vi "Control_Panel_Execute.vi"() -> ()   [LabVIEW 2019]
uses:
  Globals/Control_Panel_Globals.vi
  <vilib>/Rock Robotics/WPI/ThirdParty/REV Robotics/SPARK MAX/Typedef/Spark MAX Control Type.ctl
panel:
  in  "Positional Throttle":dbl
  in  "Color Input From Our Sensor":enum16{"Yellow", "Red", "Green", "Blue"}(ring)
  in  "time_to_run":u32
  in  "Rotational Throttle":dbl
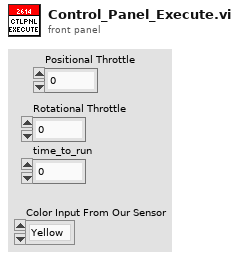
[diagram p1: front panel]
types:
  T1 = typedef "WPI_MotorControlDeviceRef.ctl" = cluster{"DeviceStatus":errorcluster, "Type":T2, "PWM":cluster{"PWM Channel":T3, "DeadBand":T4}, "CAN":cluster{"Device Number":u8, "SetOutput VI Ref":variant, "GetOutput VI Ref":variant, "Enable VI Ref":variant, "Disable VI Ref":variant, "Data":variant}, "Invert":bool, "DIO PWM":cluster{"PWM \"Enable\" Channel":T3, "DIOChannel":T5, "PWM Rate":dbl}}
  T2 = typedef "WPI_MotorControlType.ctl" = enum16{"PWM", "CAN", "DIO PWM"}
  T3 = typedef "FPGA_DIOPWMChannel.ctl" = enum8{"PWM 0", "PWM 1", "PWM 2", "PWM 3", "PWM 4", "PWM 5", "PWM 6", "PWM 7", "PWM 8", "PWM 9", "PWM MXP 0", "PWM MXP 1", "PWM MXP 2", "PWM MXP 3", "PWM MXP 4", "PWM MXP 5", "PWM MXP 6", "PWM MXP 7", "PWM MXP 8", "PWM MXP 9", "Invalid"}
  T4 = typedef "WPI_PWMDeadband.ctl" = cluster{"Name":string, "maxPositivePwm":i32, "minPositivePwm":i32, "centerPwm":i32, "maxNegativePwm":i32, "minNegativePwm":i32, "angularRange":u16}
  T5 = typedef "FPGA_DIOChannel.ctl" = enum8{"DIO 0", "DIO 1", "DIO 2", "DIO 3", "DIO 4", "DIO 5", "DIO 6", "DIO 7", "DIO 8", "DIO 9", "DIO MXP 0", "DIO MXP 1", "DIO MXP 2", "DIO MXP 3", "DIO MXP 4", "DIO MXP 5", "DIO MXP 6", "DIO MXP 7", "DIO MXP 8", "DIO MXP 9", "DIO MXP 10", "DIO MXP 11", "DIO MXP 12", "DIO MXP 13", "DIO MXP 14", "DIO MXP 15", "SPI Port CS1", "SPI Port CS2", "SPI Port CS3", "SPI Port MISO", "SPI Port MOSI", "Invalid"}
  T6 = typedef "Spark MAX Control Type.ctl" = enum16{"Percent VBus", "Voltage", "Velocity", "Position", "Smart Motion", "Current", "Smart Velocity"}
  T7 = typedef "Control_Panel_Cluster.ctl" = cluster{"Control_State":T8, "Start_Movement":bool, "Abort":bool, "Rotation_Control?":bool, "Positional_Control? ":bool, "Throttle":dbl}
  T8 = typedef "Control_Panel_States.ctl" = enum16{"No-Op", "Rotational_Control", "Positional_Control", "Manual_Control"}
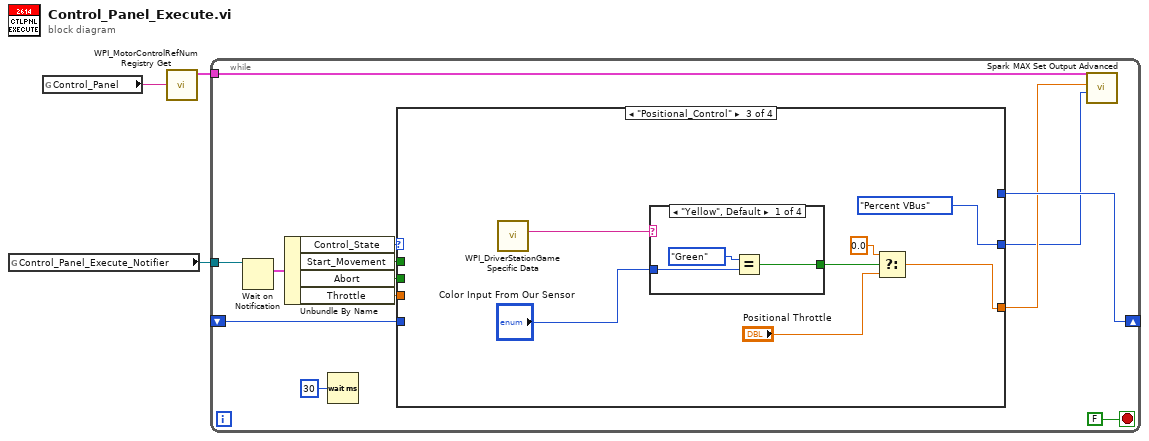
[diagram p0: block diagram]
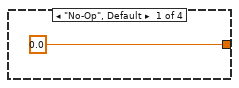
[diagram p2: hidden frame]
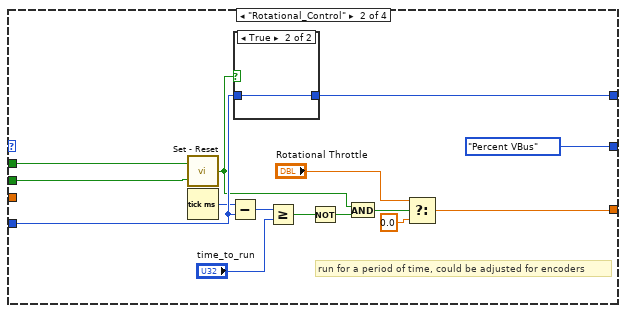
[diagram p3: hidden frame]
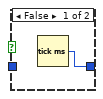
[diagram p4: hidden frame]
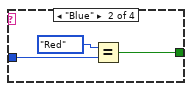
[diagram p5: hidden frame]
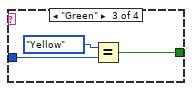
[diagram p6: hidden frame]
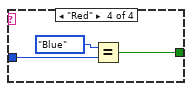
[diagram p7: hidden frame]
diagram:
  n1 = global read "Control_Panel_Globals.vi" "Control_Panel_Execute_Notifier"() -> (w3:refnum<notifier>)
  n2 = global read "Control_Panel_Globals.vi" "Control_Panel"() -> (w2:string)
  n3 = call <vilib>:"WPI_MotorControlRefNum Registry Get.vi"("refnum name"=w2) -> ("MotorControlDevRef"=w1:T1)  [unwired: 9 in, 1 out]
  n4 = while {
    tunnel: w3 -> [w16]
    shift-right: [w10] -> _
    shift-left: _ -> [w9]
    tunnel: w1 -> [w4]
    stop <- FALSE stop-if-true
    n5 = Wait on Notification(notifier=w16) -> (notification=w15:T7)  [unwired: 3 in, 3 out]
    n6 = Unbundle By Name(w15) -> ("Control_State"=w14:T8, "Start_Movement"=w12:bool, "Abort"=w11:bool, "Throttle"=w13:dbl)
    n7 = Wait (ms)(milliseconds to wait=u32 30) -> ()  [unwired: 1 out]
    n8 = case shown="\"Positional_Control\"" w14 {
      tunnel: [0.0 ("Spin_Wheel_Speed") w19 w37 w54] -> w6
      tunnel: w13 -> [_ _ _ w54]
      tunnel: w12 -> [_ w32 _ _]
      tunnel: w11 -> [_ w31 _ _]
      tunnel: [_ w29 _ _] -> w10
      tunnel: w9 -> [_ w26 _ _]
      tunnel: [_ Spark_MAX_Control_Type."Percent VBus" ("Control Mode") Spark_MAX_Control_Type."Percent VBus" ("Control Mode") _] -> w5
      frame "No-Op", Default {
      }
      frame "Rotational_Control" {
        # "run for a period of time, could be adjusted for encoders"
        n9 = call "Set - Reset.vi"("Reset"=w31, "Set"=w32) -> ("Output"=w24:bool)
        n10 = Tick Count (ms)() -> (millisecond timer value=w25:u32)
        n11 = Subtract(x=w25, y=w26) -> (x-y=w28:u32)
        n12 = case shown="True" w24 {
          tunnel: [w33 w34] -> w29
          tunnel: w26 -> [_ w34]
          frame False {
            n13 = Tick Count (ms)() -> (millisecond timer value=w33:u32)
          }
          frame True {
          }
        }
        n14 = Greater Or Equal?(x=w28, y="time_to_run") -> (x >= y?=w23:bool)
        n15 = Not(x=w23) -> (.not. x?=w22:bool)
        n16 = And(x=w24, y=w22) -> (x .and. y?=w21:bool)
        n17 = Select(t="Rotational Throttle", s=w21, f=0.0) -> (s? t:f=w19:dbl)
      }
      frame "Positional_Control" {
        n18 = call <vilib>:"WPI_DriverStationGame Specific Data.vi"() -> ("Game Specific Data"=w38:string)  [unwired: 11 in]
        n19 = case shown="\"Yellow\", Default" w38 {
          tunnel: "Color Input From Our Sensor" -> [w43 w45 w48 w51]
          tunnel: [w44 w46 w49 w52] -> w40
          frame "Yellow", Default {
            n20 = Equal?(x=enum16{"Yellow", "Red", "Green", "Blue"}."Green", y=w43) -> (x = y?=w44:bool)
          }
          frame "Blue" {
            n21 = Equal?(x=enum16{"Yellow", "Red", "Green", "Blue"}."Red", y=w45) -> (x = y?=w46:bool)
          }
          frame "Green" {
            n22 = Equal?(x=enum16{"Yellow", "Red", "Green", "Blue"}."Yellow", y=w48) -> (x = y?=w49:bool)
          }
          frame "Red" {
            n23 = Equal?(x=enum16{"Yellow", "Red", "Green", "Blue"}."Blue", y=w51) -> (x = y?=w52:bool)
          }
        }
        n24 = Select(t=0.0 ("Output"), s=w40, f="Positional Throttle") -> (s? t:f=w37:dbl)
      }
      frame "Manual_Control" {
      }
    }
    n25 = call <vilib>:"Spark MAX Set Output Advanced.vi"("Control Mode"=w5, "Setpoint"=w6, "MotorControlDevRef"=w4) -> ()  [unwired: 7 in, 2 out]
  }
